vi "DAD.vi"(7 "DRIVER STOP":bool, 8 "BAD DOWN":bool, 9 "BAD UP":bool, 10 "BAD OUT":bool, 11 "BAD IN":bool) -> (3 "BAD On?":bool)   [LabVIEW 2012]
uses:
  <vilib>/Rock Robotics/WPI/Relay/WPI_RelayValue.ctl
  Robot Global Data.vi
  <vilib>/Rock Robotics/WPI/Solenoid/Deprecated/WPI_SolenoidSetBool.vi
panel:
  out "BAD Output":T1
  # "For debugging, later use constant"
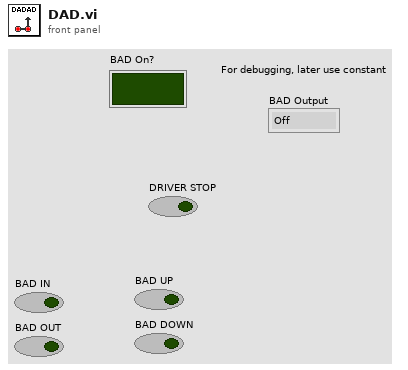
[diagram p1: front panel]
types:
  T1 = typedef "WPI_RelayValue.ctl" = enum16{"Off", "On", "Forward", "Reverse"}
  T2 = typedef "WPI_SolenoidDevRef.ctl" = cluster{"DevStatus":errorcluster, "Solenoid Module":T3, "Forward Solenoid Channel":T4, "Reverse Solenoid Channel":T4}
  T3 = typedef "FPGA_TypedefSolenoidModule.ctl" = enum16{"Solenoid Module 1", "Solenoid Module 2"}
  T4 = typedef "WPI_SolenoidChannel.ctl" = enum8{"Solenoid 1", "Solenoid 2", "Solenoid 3", "Solenoid 4", "Solenoid 5", "Solenoid 6", "Solenoid 7", "Solenoid 8", "Invalid"}
  T5 = typedef "WPI_RelayDevRef.ctl" = cluster{"DevStatus":errorcluster, "Relay Channel":T6, "Digital Module":T7, "Relay Direction":T8}
  T6 = typedef "FPGA_DIORelayChannel.ctl" = enum8{"Relay 1", "Relay 2", "Relay 3", "Relay 4", "Relay 5", "Relay 6", "Relay 7", "Relay 8", "Invalid"}
  T7 = typedef "FPGA_TypedefDigitalModule.ctl" = enum16{"Digital Module 1", "Digital Module 2"}
  T8 = typedef "WPI_RelayDirection.ctl" = enum16{"Both directions", "Forward only", "Reverse only"}
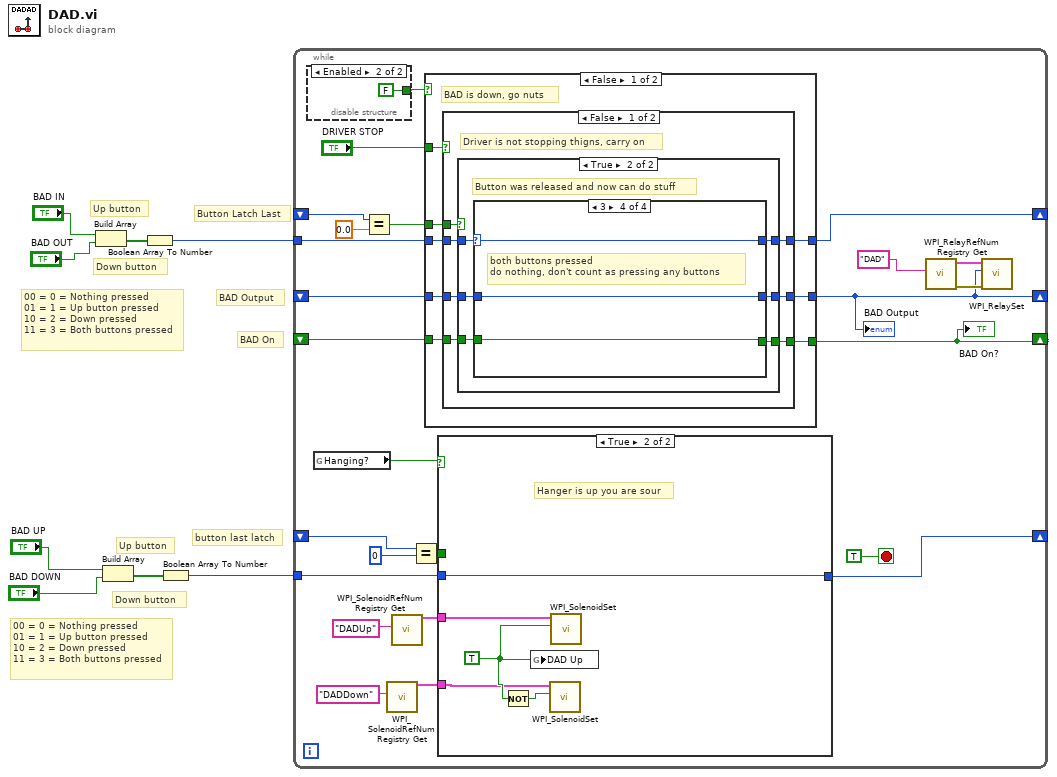
[diagram p0: block diagram]
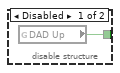
[diagram p2: hidden frame]
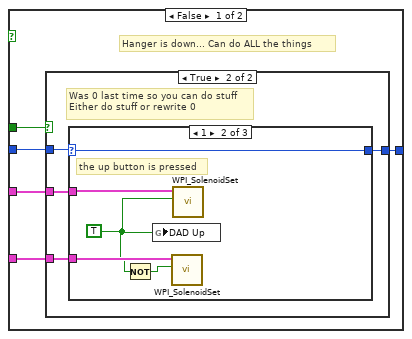
[diagram p3: hidden frame]
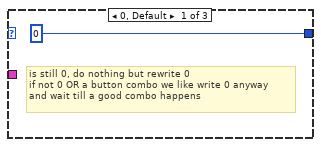
[diagram p5: hidden frame]
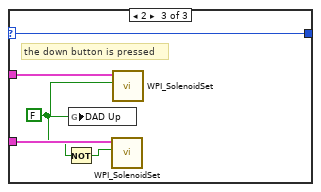
[diagram p6: hidden frame]
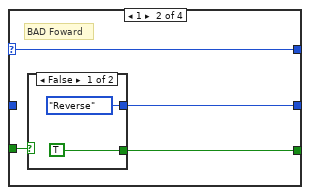
[diagram p9: hidden frame]
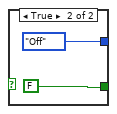
[diagram p10: hidden frame]
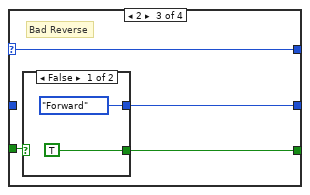
[diagram p11: hidden frame]
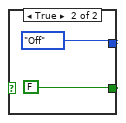
[diagram p12: hidden frame]
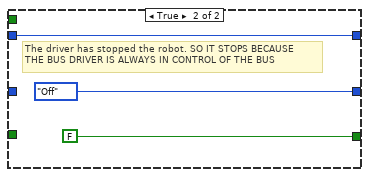
[diagram p13: hidden frame]
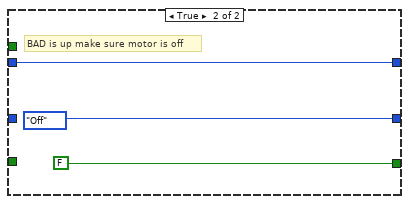
[diagram p14: hidden frame]
diagram:
  # "button last latch"
  # "Button Latch Last"
  # "BAD On"
  # "BAD Output"
  # "Down button"
  # "Up button"
  # "00 = 0 = Nothing pressed\n01 = 1 = Up button pressed\n10 = 2 = Down pressed\n11 = 3 = Both buttons pressed"
  # "Down button"
  # "Up button"
  # "00 = 0 = Nothing pressed\n01 = 1 = Up button pressed\n10 = 2 = Down pressed\n11 = 3 = Both buttons pressed"
  n1 = Build Array("BAD IN", "BAD OUT") -> (w8:bool[])
  n2 = Build Array("BAD UP", "BAD DOWN") -> (w7:bool[])
  n3 = Boolean Array To Number(Boolean array=w8) -> (number=w1:u32)
  n4 = Boolean Array To Number(Boolean array=w7) -> (number=w6:u32)
  n5 = while {
    tunnel: w6 -> [w30]
    tunnel: w1 -> [w25]
    shift-right: [w20] -> _
    shift-left: _ -> [w15]
    shift-right: [w19] -> _
    shift-left: _ -> [w18]
    shift-right: [w17] -> _
    shift-left: _ -> [w16]
    shift-right: [w14] -> _
    shift-left: _ -> [w13]
    stop <- TRUE stop-if-true
    n6 = disable-structure shown="Enabled" {
      disable-tunnel: [w34 FALSE ("DAD Up")] -> w27
      frame Disabled {
        n7 = global read "Robot Global Data.vi" "DAD Up"() -> (w34:bool)
      }
      frame Enabled {
      }
    }
    n8 = global read "Robot Global Data.vi" "Hanging?"() -> (w9:bool)
    n9 = Equal?(x=w16, y=0.0) -> (x = y?=w33:bool)
    n10 = call <vilib>:"WPI_SolenoidRefNum Registry Get.vi"("refnum name"="DADDown") -> ("SolenoidDevRef"=w28:T2)  [unwired: 9 in, 1 out]
    n11 = call <vilib>:"WPI_SolenoidRefNum Registry Get.vi"("refnum name"="DADUp") -> ("SolenoidDevRef"=w29:T2)  [unwired: 9 in, 1 out]
    n12 = Equal?(x=w13, y=0) -> (x = y?=w32:bool)
    n13 = case shown="False" w27 {
      tunnel: w33 -> [w69 _]
      tunnel: w25 -> [w68 w111]
      tunnel: "DRIVER STOP" -> [w67 _]
      tunnel: [w66 WPI_RelayValue."Off" ("BAD Output")] -> w20
      tunnel: [w65 FALSE] -> w19
      tunnel: w18 -> [w64 _]
      tunnel: [w63 w111] -> w17
      tunnel: w15 -> [w62 _]
      frame False {
        # "BAD is down, go nuts"
        n14 = case shown="False" w67 {
          tunnel: w69 -> [w76 _]
          tunnel: w68 -> [w75 w108]
          tunnel: [w74 WPI_RelayValue."Off" ("BAD Output")] -> w66
          tunnel: [w73 FALSE] -> w65
          tunnel: w64 -> [w72 _]
          tunnel: [w71 w108] -> w63
          tunnel: w62 -> [w70 _]
          frame False {
            # "Driver is not stopping thigns, carry on"
            n15 = case shown="True" w76 {
              tunnel: w75 -> [w79 w85]
              tunnel: [w78 w84] -> w74
              tunnel: [w77 w83] -> w73
              tunnel: w72 -> [w77 w82]
              tunnel: [w79 w81] -> w71
              tunnel: w70 -> [w78 w80]
              frame False {
                # "Hasn't been released yet, don't do anything\nrecord value so it can be 0 (or not) next loop"
              }
              frame True {
                # "Button was released and now can do stuff"
                n16 = case shown="3" w85 {
                  selector: w85 -> [w88 w92 w97 w105]
                  tunnel: [w87 w91 w100 w107] -> w84
                  tunnel: [w86 w90 w99 w106] -> w83
                  tunnel: w82 -> [w86 w89 w98 w106]
                  tunnel: [w88 w92 w97 w105] -> w81
                  tunnel: w80 -> [w87 _ _ w107]
                  frame 0, Default {
                    # "no buttons pressed\ndo nothing"
                  }
                  frame 1 {
                    # "BAD Foward"
                    n17 = case shown="False" w89 {
                      tunnel: [WPI_RelayValue."Reverse" ("BAD Output") WPI_RelayValue."Off" ("BAD Output")] -> w91
                      tunnel: [TRUE FALSE] -> w90
                      frame False {
                      }
                      frame True {
                      }
                    }
                  }
                  frame 2 {
                    # "Bad Reverse"
                    n18 = case shown="False" w98 {
                      tunnel: [WPI_RelayValue."Forward" ("BAD Output") WPI_RelayValue."Off" ("BAD Output")] -> w100
                      tunnel: [TRUE FALSE] -> w99
                      frame False {
                      }
                      frame True {
                      }
                    }
                  }
                  frame 3 {
                    # "both buttons pressed\ndo nothing, don't count as pressing any buttons"
                  }
                }
              }
            }
          }
          frame True {
            # "The driver has stopped the robot. SO IT STOPS BECAUSE\nTHE BUS DRIVER IS ALWAYS IN CONTROL OF THE BUS"
          }
        }
      }
      frame True {
        # "BAD is up make sure motor is off"
      }
    }
    "BAD On?" <- w19
    "BAD Output" <- w20
    n19 = case shown="True" w9 {
      tunnel: w32 -> [w40 _]
      tunnel: w30 -> [w39 w57]
      tunnel: w29 -> [w38 w59]
      tunnel: w28 -> [w37 w58]
      tunnel: [w36 w57] -> w14
      frame False {
        # "Hanger is down... Can do ALL the things"
        n20 = case shown="True" w40 {
          tunnel: w39 -> [w41 w45]
          tunnel: w38 -> [_ w44]
          tunnel: w37 -> [_ w43]
          tunnel: [w41 w42] -> w36
          frame False {
            # "Write the current state waiting for it to be 0"
          }
          frame True {
            # "Was 0 last time so you can do stuff\nEither do stuff or rewrite 0"
            n21 = case shown="1" w45 {
              selector: w45 -> [_ w48 w53]
              tunnel: w44 -> [_ w51 w56]
              tunnel: w43 -> [_ w50 w55]
              tunnel: [0 w48 w53] -> w42
              frame 0, Default {
                # "is still 0, do nothing but rewrite 0\nif not 0 OR a button combo we like write 0 anyway\nand wait till a good combo happens"
              }
              frame 1 {
                w47 = TRUE
                # "the up button is pressed"
                n22 = Not(x=w47) -> (.not. x?=w49:bool)
                n23 = global write "Robot Global Data.vi" "DAD Up"(w47) -> ()
                n24 = call-poly <vilib>:"WPI_SolenoidSet.vi"("Value"=w49, "SolenoidDevRef"=w50) -> ()  [unwired: 8 in, 2 out]
                n25 = call-poly <vilib>:"WPI_SolenoidSet.vi"("Value"=w47, "SolenoidDevRef"=w51) -> ()  [unwired: 8 in, 2 out]
              }
              frame 2 {
                w52 = FALSE
                # "the down button is pressed"
                n26 = Not(x=w52) -> (.not. x?=w54:bool)
                n27 = global write "Robot Global Data.vi" "DAD Up"(w52) -> ()
                n28 = call-poly <vilib>:"WPI_SolenoidSet.vi"("Value"=w54, "SolenoidDevRef"=w55) -> ()  [unwired: 8 in, 2 out]
                n29 = call-poly <vilib>:"WPI_SolenoidSet.vi"("Value"=w52, "SolenoidDevRef"=w56) -> ()  [unwired: 8 in, 2 out]
              }
            }
          }
        }
      }
      frame True {
        w60 = TRUE
        # "Hanger is up you are sour"
        n30 = Not(x=w60) -> (.not. x?=w61:bool)
        n31 = global write "Robot Global Data.vi" "DAD Up"(w60) -> ()
        n32 = call-poly <vilib>:"WPI_SolenoidSet.vi"("Value"=w61, "SolenoidDevRef"=w58) -> ()  [unwired: 8 in, 2 out]
        n33 = call-poly <vilib>:"WPI_SolenoidSet.vi"("Value"=w60, "SolenoidDevRef"=w59) -> ()  [unwired: 8 in, 2 out]
      }
    }
    n34 = call <vilib>:"WPI_RelayRefNum Registry Get.vi"("refnum name"="DAD") -> ("error out"=w23:errorcluster, "RelayDevRef"=w22:T5)  [unwired: 9 in]
    n35 = call <vilib>:"WPI_RelaySet.vi"("error in (no error)"=w23, "RelayValue"=w20, "RelayDevRef"=w22) -> ()  [unwired: 7 in, 2 out]
  }
